vi "HFRR ADV v036 new software.vi"() -> ()   [LabVIEW 2025] (continued)
            n1884 = local write "Main Tab"(T2."Advance" ("Main Tab")) -> ()
            n1885 = local write "Main Dashboard Buttons"(T1."Advance" ("Main Dashboard Buttons")) -> ()
          }
        }
      }
    }
    n1886 = case shown="True" "Prog Uno" {
      frame False {
      }
      frame True {
        n1887 = stacked-sequence {
          frame #0 {
            n1888 = Delete(path (use dialog)=path "C:/LAB-IQ-NXT/UNOCOMPILE.bat" ("working directory")) -> ()  [unwired: 4 in, 3 out]
          }
          frame #1 {
            n1889 = local read "Com Port 1"() -> (w2647:refnum<visa-resource-name>)
            n1890 = Concatenate Strings("cmd.exe /c \"mode " ("command line"), w2647, ":1200,n,8,1\"\n" ("command line")) -> (w2652:string)
            n1891 = Concatenate Strings(w2652, "CD\\\nCD WinDucom\navrdude -C avrdude.conf -v -patmega328p -carduino -P" ("command line"), w2647, " -b115200 -D -Uflash:w:UNO_V20.hex:i\n" ("command line"), "\r") -> (w2654:string)
            "STR" <- w2654
            n1892 = call <vilib>:"Write Characters To File.vi"("append to file? (new file:F)"=FALSE, "character string"=w2654, "file path (dialog if empty)"=path "C:/LAB-IQ/UNOCOMPILE.bat" ("working directory")) -> ()  [unwired: 2 in, 1 out]
          }
          frame #2 {
            n1893 = disable-structure shown="Disabled" {
              frame Disabled {
                w2658 = "cmd.exe  /c \"C:\\LAB-IQ-NXT\\UNOCOMPILE.bat\"" ("string")
                n1894 = local write "Prog Uno"(FALSE ("run minimized? (F)")) -> ()
                n1895 = call <vilib>:"System Exec.vi"("expected output size  (4096)"=u32 65535, "run minimized? (F)"=FALSE, "wait until completion? (T)"=TRUE ("run minimized? (F)"), "working directory"=path "C:/LAB-IQ-NXT", "standard input"=w2658, "command line"=w2658) -> ("error out"=w2657:errorcluster, "standard output"=→"String 42":string)  [unwired: 2 in, 2 out]
                "error out 3" <- w2657
                n1896 = flat-sequence {
                  tunnel: w2657 -> [_]
                  frame #0 {
                  }
                }
              }
              frame Enabled {
              }
            }
          }
        }
      }
    }
    n1897 = case shown="\"ISO 12156\"" "TEST STANDARD" {
      frame "ASTM D6079", Default {
        w2627 = 50.0 ("Hz")
        w2628 = 53.0 ("Set Rh")
        w2630 = 1.0 ("Set Strk")
        w2629 = 60.0 ("Set Temp")
        # "astm hide"
        n1898 = local write "NORMAL LOAD"(200.0 ("NORMAL LOAD")) -> ()
        n1899 = local write "Set Strk"(w2630) -> ()
        n1900 = local write "Set Hz"(w2627) -> ()
        n1901 = local write "Set Temp"(w2629) -> ()
        n1902 = local write "Set Rh"(w2628) -> ()
        n1903 = local write "test time"(75.0 ("test time")) -> ()
        n1904 = local write "Set Stroke:"(w2630) -> ()
        n1905 = local write "Set Humidity:"(w2628) -> ()
        n1906 = local write "Set Frequency:"(w2627) -> ()
        n1907 = local write "Set Temperature:"(w2629) -> ()
        "Test Standard" <- "ASTM D6079" ("Test Standard 2")
      }
      frame "ISO 12156" {
        n1908 = local write "Set Strk"(1.0 ("Set Strk")) -> ()
        n1909 = local write "NORMAL LOAD"(200.0 ("NORMAL LOAD")) -> ()
        n1910 = local write "Set Temp"(60.0 ("Set Temp")) -> ()
        n1911 = local write "test time"(75.0 ("test time")) -> ()
        n1912 = local write "Set Hz"(50.0 ("Hz")) -> ()
        n1913 = local write "Set Rh"(53.0 ("Set Rh")) -> ()
      }
      frame "CEC F-096-A-06" {
        n1914 = local write "Set Strk"(1.0 ("Set Strk")) -> ()
        n1915 = local write "NORMAL LOAD"(200.0 ("NORMAL LOAD")) -> ()
        n1916 = local write "Set Temp"(60.0 ("Set Temp")) -> ()
        n1917 = local write "test time"(75.0 ("test time")) -> ()
        n1918 = local write "Set Hz"(50.0 ("Hz")) -> ()
        n1919 = local write "Set Rh"(53.0 ("Set Rh")) -> ()
      }
      frame "Custom" {
      }
    }
    n1920 = Or(x=w2180, y=w2178) -> (x .or. y?=w2179:bool)
    n1921 = case shown="\"About\"" w2177 {
      tunnel: [T28."Acquire" ("Main Tab") T28."Compare Files" ("Main Tab") T28."About" ("Main Tab")] -> w2188
      frame "Acquire", Default {
      }
      frame "Compare Files" {
      }
      frame "About" {
      }
    }
    n1922 = Or(x=w2183, y="OPEN") -> (x .or. y?=w2184:bool)
    n1923 = case shown="True" w2184 {
      tunnel: w2183 -> [_ w2216]
      frame False {
      }
      frame True {
        n1924 = stacked-sequence {
          tunnel: w2216 -> [_ w2283 _ _]
          frame #0 {
            w2232 = "  " ("String 6")
            n1925 = local write "OPEN"(FALSE ("open")) -> ()
            n1926 = local read "string1 2"() -> (w2220:string)
            n1927 = local read "string1 3"() -> (w2219:string)
            n1928 = local read "string1 4"() -> (w2218:string)
            n1929 = property on="OPEN" class="Bool (strict)"("Visible"=FALSE) -> ()  [unwired: 2 in, 2 out]
            n1930 = local write "String 6"(w2232) -> ()
            n1931 = local write "String 7"(w2232) -> ()
            n1932 = local write "String 8"(w2232) -> ()
            n1933 = local write "String 12"(w2232) -> ()
            n1934 = local read "OK Button 16"() -> (w2217:bool)
            n1935 = String To Path(string=w2220) -> (path=w2228:path)
            n1936 = String To Path(string=w2219) -> (path=w2227:path)
            n1937 = String To Path(string=w2218) -> (path=w2226:path)
            n1938 = case shown="True" w2217 {
              tunnel: [w2233 w2234] -> w2221
              frame False {
                n1939 = local read "string1"() -> (w2233:string)
              }
              frame True {
                n1940 = local read "String Indicator 4"() -> (w2234:string)
              }
            }
            n1941 = Open/Create/Replace File "Open File"(file path (use dialog)=w2228) -> (refnum out=w2224:refnum<file>)  [unwired: 5 in, 2 out]
            n1942 = Open/Create/Replace File "Open File"(file path (use dialog)=w2227) -> (refnum out=w2223:refnum<file>)  [unwired: 5 in, 2 out]
            n1943 = Open/Create/Replace File "Open File"(file path (use dialog)=w2226) -> (refnum out=w2222:refnum<file>)  [unwired: 5 in, 2 out]
            n1944 = while {
              tunnel: w2224 -> [w2246]
              i -> [w2242]
              stop <- w2241 continue-if-true
              (unwired) TRUE ("line mode (F)")
              n1945 = Read from Text File "Read File"(file (use dialog)=w2246) -> (text=w2243:string)  [unwired: 3 in, 3 out]
              n1946 = local write "Numeric 11"(w2242) -> ()
              n1947 = String Length(string=w2243) -> (length=w2245:i32)
              n1948 = Greater?(x=w2245, y=1) -> (0:w2241:bool)
            }
            n1949 = while {
              tunnel: w2223 -> [w2252]
              i -> [w2248]
              stop <- w2247 continue-if-true
              (unwired) TRUE ("line mode (F)")
              n1950 = Read from Text File "Read File"(file (use dialog)=w2252) -> (text=w2249:string)  [unwired: 3 in, 3 out]
              n1951 = local write "Numeric 12"(w2248) -> ()
              n1952 = String Length(string=w2249) -> (length=w2251:i32)
              n1953 = Greater?(x=w2251, y=1) -> (0:w2247:bool)
            }
            n1954 = while {
              tunnel: w2222 -> [w2258]
              i -> [w2254]
              stop <- w2253 continue-if-true
              (unwired) TRUE ("line mode (F)")
              n1955 = Read from Text File "Read File"(file (use dialog)=w2258) -> (text=w2255:string)  [unwired: 3 in, 3 out]
              n1956 = local write "Numeric 13"(w2254) -> ()
              n1957 = String Length(string=w2255) -> (length=w2257:i32)
              n1958 = Greater?(x=w2257, y=1) -> (0:w2253:bool)
            }
            n1959 = String To Path(string=w2221) -> (path=w2229:path)
            n1960 = Open/Create/Replace File "Open File"(file path (use dialog)=w2229) -> (refnum out=w2225:refnum<file>)  [unwired: 5 in, 2 out]
            n1961 = while {
              tunnel: w2225 -> [w2240]
              i -> [w2236]
              stop <- w2235 continue-if-true
              (unwired) TRUE ("line mode (F)")
              n1962 = Read from Text File "Read File"(file (use dialog)=w2240) -> (text=w2237:string)  [unwired: 3 in, 3 out]
              n1963 = local write "Numeric 8"(w2236) -> ()
              n1964 = String Length(string=w2237) -> (length=w2239:i32)
              n1965 = Greater?(x=w2239, y=1) -> (0:w2235:bool)
            }
          }
          frame #1 {
            w2410 = FALSE ("ACTUAL   MERGE")
            # "Sample Temp"
            # "ECR"
            # "COF"
            # "Time\nCOF\nFF\nTemp"
            n1966 = case shown="True" w2283 {
              tunnel: [w2430 w2431] -> w2284
              frame False {
                n1967 = local read "string1"() -> (w2430:string)
              }
              frame True {
                n1968 = local read "String Indicator 4"() -> (w2431:string)
              }
            }
            n1969 = local read "string1 3"() -> (w2328:string)
            n1970 = String To Path(string=w2284) -> (path=w2415:path)
            n1971 = String To Path(string=w2328) -> (path=w2426:path)
            n1972 = local read "Numeric 12"() -> (w2412:i32)
            n1973 = local read "Numeric 8"() -> (w2414:i32)
            n1974 = local read "string1 2"() -> (w2329:string)
            n1975 = local read "string1 4"() -> (w2327:string)
            n1976 = Open/Create/Replace File "Open File"(file path (use dialog)=w2415) -> (refnum out=w2429:refnum<file>, error out=w2428:errorcluster)  [unwired: 5 in, 1 out]
            n1977 = Open/Create/Replace File "Open File"(file path (use dialog)=w2426) -> (refnum out=w2422:refnum<file>, error out=w2423:errorcluster)  [unwired: 5 in, 1 out]
            n1978 = for {
              N: w2414 -> [_]
              tunnel: w2429 -> [w2577]
              tunnel: w2428 -> [w2576]
              tunnel: [w2566] -> w2341 mode=indexing
              tunnel: [w2564] -> w2398 mode=indexing
              tunnel: [w2565] -> w2393 mode=indexing
              tunnel: w2410 -> [_]
              tunnel: [w2558] -> w2395 mode=indexing
              tunnel: [w2554] -> w2364 mode=indexing
              tunnel: [w2550] -> w2339 mode=indexing
              tunnel: [w2546] -> w2320 mode=indexing
              tunnel: [w2541] -> w2280 mode=indexing
              (unwired) TRUE ("line mode (F)")
              # "freq"
              # "Stroke"
              # "Time"
              # "CoF"
              # "Humidity"
              # "Temp"
              # "Air Temp"
              # "ECR"
              n1979 = Read from Text File "Read File"(file (use dialog)=w2577, error in=w2576) -> (text=w2542:string)  [unwired: 2 in, 3 out]
              n1980 = local write "String 6"(w2542) -> ()
              n1981 = String Subset(string=w2542, offset (0)=0, length (rest)=14 ("length (rest)")) -> (substring=w2570:string)
              n1982 = String Subset(string=w2542, offset (0)=35, length (rest)=9 ("length (rest)")) -> (substring=w2567:string)
              n1983 = String Subset(string=w2542, offset (0)=15, length (rest)=9 ("length (rest)")) -> (substring=w2573:string)
              n1984 = Fract/Exp String To Number(string=w2570) -> (number=w2566:dbl)  [unwired: 3 in, 1 out]
              n1985 = Fract/Exp String To Number(string=w2567) -> (number=w2565:dbl)  [unwired: 3 in, 1 out]
              n1986 = Fract/Exp String To Number(string=w2573) -> (number=w2564:dbl)  [unwired: 3 in, 1 out]
              n1987 = String Subset(string=w2542, offset (0)=85, length (rest)=9 ("length (rest)")) -> (substring=w2543:string)
              n1988 = String Subset(string=w2542, offset (0)=25, length (rest)=9 ("length (rest)")) -> (substring=w2549:string)
              n1989 = String Subset(string=w2542, offset (0)=55, length (rest)=9 ("length (rest)")) -> (substring=w2551:string)
              n1990 = String Subset(string=w2542, offset (0)=45, length (rest)=9 ("length (rest)")) -> (substring=w2557:string)
              n1991 = String Subset(string=w2542, offset (0)=65, length (rest)=9 ("length (rest)")) -> (substring=w2563:string)
              n1992 = Fract/Exp String To Number(string=w2549) -> (number=w2546:dbl)  [unwired: 3 in, 1 out]
              n1993 = Fract/Exp String To Number(string=w2543) -> (number=w2541:dbl)  [unwired: 3 in, 1 out]
              n1994 = Fract/Exp String To Number(string=w2551) -> (number=w2550:dbl)  [unwired: 3 in, 1 out]
              n1995 = Fract/Exp String To Number(string=w2557) -> (number=w2554:dbl)  [unwired: 3 in, 1 out]
              n1996 = Fract/Exp String To Number(string=w2563) -> (number=w2560:dbl)  [unwired: 3 in, 1 out]
              n1997 = Add(x=w2560, y=0.0) -> (x+y=w2558:dbl)
            }
            n1998 = for {
              N: w2412 -> [_]
              tunnel: w2423 -> [w2503]
              tunnel: w2422 -> [w2502]
              tunnel: [w2492] -> w2381 mode=indexing
              tunnel: [w2490] -> w2379 mode=indexing
              tunnel: [w2491] -> w2375 mode=indexing
              tunnel: w2410 -> [_]
              tunnel: [w2484] -> w2377 mode=indexing
              tunnel: [w2480] -> w2359 mode=indexing
              tunnel: [w2476] -> w2335 mode=indexing
              tunnel: [w2473] -> w2316 mode=indexing
              tunnel: [w2469] -> w2275 mode=indexing
              (unwired) 9 ("length (rest)")
              (unwired) 9 ("length (rest)")
              (unwired) TRUE ("line mode (F)")
              n1999 = Read from Text File "Read File"(file (use dialog)=w2502, error in=w2503) -> (text=w2470:string)  [unwired: 2 in, 3 out]
              n2000 = local write "String 8"(w2470) -> ()
              n2001 = String Subset(string=w2470, offset (0)=85) -> (substring=w2472:string)  [unwired: 1 in]
              n2002 = String Subset(string=w2470, offset (0)=35, length (rest)=9 ("length (rest)")) -> (substring=w2493:string)
              n2003 = String Subset(string=w2470, offset (0)=55, length (rest)=9 ("length (rest)")) -> (substring=w2478:string)
              n2004 = String Subset(string=w2470, offset (0)=25) -> (substring=w2474:string)  [unwired: 1 in]
              n2005 = String Subset(string=w2470, offset (0)=15, length (rest)=9 ("length (rest)")) -> (substring=w2499:string)
              n2006 = String Subset(string=w2470, offset (0)=0, length (rest)=14 ("length (rest)")) -> (substring=w2496:string)
              n2007 = String Subset(string=w2470, offset (0)=45, length (rest)=9 ("length (rest)")) -> (substring=w2483:string)
              n2008 = String Subset(string=w2470, offset (0)=65, length (rest)=9 ("length (rest)")) -> (substring=w2489:string)
              n2009 = Fract/Exp String To Number(string=w2472) -> (number=w2469:dbl)  [unwired: 3 in, 1 out]
              n2010 = Fract/Exp String To Number(string=w2493) -> (number=w2491:dbl)  [unwired: 3 in, 1 out]
              n2011 = Fract/Exp String To Number(string=w2478) -> (number=w2476:dbl)  [unwired: 3 in, 1 out]
              n2012 = Fract/Exp String To Number(string=w2474) -> (number=w2473:dbl)  [unwired: 3 in, 1 out]
              n2013 = Fract/Exp String To Number(string=w2499) -> (number=w2490:dbl)  [unwired: 3 in, 1 out]
              n2014 = Fract/Exp String To Number(string=w2496) -> (number=w2492:dbl)  [unwired: 3 in, 1 out]
              n2015 = Fract/Exp String To Number(string=w2483) -> (number=w2480:dbl)  [unwired: 3 in, 1 out]
              n2016 = Fract/Exp String To Number(string=w2489) -> (number=w2486:dbl)  [unwired: 3 in, 1 out]
              n2017 = Add(x=w2486, y=0.0) -> (x+y=w2484:dbl)
            }
            n2018 = String To Path(string=w2329) -> (path=w2427:path)
            n2019 = String To Path(string=w2327) -> (path=w2421:path)
            n2020 = local read "Numeric 11"() -> (w2411:i32)
            n2021 = local read "Numeric 13"() -> (w2413:i32)
            n2022 = Open/Create/Replace File "Open File"(file path (use dialog)=w2427) -> (refnum out=w2425:refnum<file>, error out=w2424:errorcluster)  [unwired: 5 in, 1 out]
            n2023 = Open/Create/Replace File "Open File"(file path (use dialog)=w2421) -> (refnum out=w2420:refnum<file>, error out=w2419:errorcluster)  [unwired: 5 in, 1 out]
            n2024 = for {
              N: w2411 -> [_]
              tunnel: w2425 -> [w2540]
              tunnel: w2424 -> [w2539]
              tunnel: [w2529] -> w2391 mode=indexing
              tunnel: [w2527] -> w2389 mode=indexing
              tunnel: [w2528] -> w2384 mode=indexing
              tunnel: w2410 -> [_]
              tunnel: [w2521] -> w2386 mode=indexing
              tunnel: [w2517] -> w2362 mode=indexing
              tunnel: [w2513] -> w2337 mode=indexing
              tunnel: [w2509] -> w2318 mode=indexing
              tunnel: [w2504] -> w2276 mode=indexing
              (unwired) TRUE ("line mode (F)")
              n2025 = Read from Text File "Read File"(file (use dialog)=w2540, error in=w2539) -> (text=w2505:string)  [unwired: 2 in, 3 out]
              n2026 = local write "String 7"(w2505) -> ()
              n2027 = String Subset(string=w2505, offset (0)=85, length (rest)=9 ("length (rest)")) -> (substring=w2508:string)
              n2028 = String Subset(string=w2505, offset (0)=35, length (rest)=9 ("length (rest)")) -> (substring=w2530:string)
              n2029 = String Subset(string=w2505, offset (0)=55, length (rest)=9 ("length (rest)")) -> (substring=w2516:string)
              n2030 = String Subset(string=w2505, offset (0)=25, length (rest)=9 ("length (rest)")) -> (substring=w2510:string)
              n2031 = String Subset(string=w2505, offset (0)=45, length (rest)=9 ("length (rest)")) -> (substring=w2518:string)
              n2032 = String Subset(string=w2505, offset (0)=0, length (rest)=14 ("length (rest)")) -> (substring=w2533:string)
              n2033 = String Subset(string=w2505, offset (0)=15, length (rest)=9 ("length (rest)")) -> (substring=w2536:string)
              n2034 = String Subset(string=w2505, offset (0)=65, length (rest)=9 ("length (rest)")) -> (substring=w2522:string)
              n2035 = Fract/Exp String To Number(string=w2508) -> (number=w2504:dbl)  [unwired: 3 in, 1 out]
              n2036 = Fract/Exp String To Number(string=w2530) -> (number=w2528:dbl)  [unwired: 3 in, 1 out]
              n2037 = Fract/Exp String To Number(string=w2516) -> (number=w2513:dbl)  [unwired: 3 in, 1 out]
              n2038 = Fract/Exp String To Number(string=w2510) -> (number=w2509:dbl)  [unwired: 3 in, 1 out]
              n2039 = Fract/Exp String To Number(string=w2518) -> (number=w2517:dbl)  [unwired: 3 in, 1 out]
              n2040 = Fract/Exp String To Number(string=w2533) -> (number=w2529:dbl)  [unwired: 3 in, 1 out]
              n2041 = Fract/Exp String To Number(string=w2536) -> (number=w2527:dbl)  [unwired: 3 in, 1 out]
              n2042 = Fract/Exp String To Number(string=w2522) -> (number=w2525:dbl)  [unwired: 3 in, 1 out]
              n2043 = Add(x=w2525, y=0.0) -> (x+y=w2521:dbl)
            }
            n2044 = for {
              N: w2413 -> [_]
              tunnel: w2420 -> [w2468]
              tunnel: w2419 -> [w2467]
              tunnel: [w2457] -> w2373 mode=indexing
              tunnel: [w2456] -> w2366 mode=indexing
              tunnel: w2410 -> [_]
              tunnel: [w2445] -> w2371 mode=indexing
              tunnel: [w2450] -> w2368 mode=indexing
              tunnel: [w2446] -> w2358 mode=indexing
              tunnel: [w2441] -> w2333 mode=indexing
              tunnel: [w2437] -> w2314 mode=indexing
              tunnel: [w2432] -> w2274 mode=indexing
              (unwired) 1.0 ("x")
              (unwired) TRUE ("line mode (F)")
              n2045 = Read from Text File "Read File"(file (use dialog)=w2468, error in=w2467) -> (text=w2433:string)  [unwired: 2 in, 3 out]
              n2046 = local write "String 12"(w2433) -> ()
              n2047 = String Subset(string=w2433, offset (0)=85, length (rest)=9 ("length (rest)")) -> (substring=w2435:string)
              n2048 = String Subset(string=w2433, offset (0)=35, length (rest)=9 ("length (rest)")) -> (substring=w2458:string)
              n2049 = String Subset(string=w2433, offset (0)=55, length (rest)=9 ("length (rest)")) -> (substring=w2443:string)
              n2050 = String Subset(string=w2433, offset (0)=25, length (rest)=9 ("length (rest)")) -> (substring=w2439:string)
              n2051 = String Subset(string=w2433, offset (0)=45, length (rest)=9 ("length (rest)")) -> (substring=w2448:string)
              n2052 = String Subset(string=w2433, offset (0)=15, length (rest)=9 ("length (rest)")) -> (substring=w2464:string)
              n2053 = String Subset(string=w2433, offset (0)=0, length (rest)=14 ("length (rest)")) -> (substring=w2461:string)
              n2054 = String Subset(string=w2433, offset (0)=65, length (rest)=9 ("length (rest)")) -> (substring=w2451:string)
              n2055 = Fract/Exp String To Number(string=w2435) -> (number=w2432:dbl)  [unwired: 3 in, 1 out]
              n2056 = Fract/Exp String To Number(string=w2458) -> (number=w2456:dbl)  [unwired: 3 in, 1 out]
              n2057 = Fract/Exp String To Number(string=w2443) -> (number=w2441:dbl)  [unwired: 3 in, 1 out]
              n2058 = Fract/Exp String To Number(string=w2439) -> (number=w2437:dbl)  [unwired: 3 in, 1 out]
              n2059 = Fract/Exp String To Number(string=w2448) -> (number=w2446:dbl)  [unwired: 3 in, 1 out]
              n2060 = Fract/Exp String To Number(string=w2464) -> (number=w2445:dbl)  [unwired: 3 in, 1 out]
              n2061 = Fract/Exp String To Number(string=w2461) -> (number=w2457:dbl)  [unwired: 3 in, 1 out]
              n2062 = Fract/Exp String To Number(string=w2451) -> (number=w2454:dbl)  [unwired: 3 in, 1 out]
              n2063 = Add(x=w2454, y=0.0) -> (x+y=w2450:dbl)
            }
            n2064 = Delete From Array(array=w2316, index=0) -> (array with subset deleted=w2289:dbl[])  [unwired: 1 in, 1 out]
            n2065 = Delete From Array(array=w2379, index=0) -> (array with subset deleted=w2352:dbl[])  [unwired: 1 in, 1 out]
            n2066 = Delete From Array(array=w2359, index=0) -> (array with subset deleted=w2347:dbl[])  [unwired: 1 in, 1 out]
            n2067 = Delete From Array(array=w2377, index=0) -> (array with subset deleted=w2378:dbl[])  [unwired: 1 in, 1 out]
            n2068 = call-poly <vilib>:"Mean.vi"("X"=w2289) -> ("mean"=→"КОФ2 4":dbl)  [unwired: 1 out]
            n2069 = call-poly <vilib>:"Mean.vi"("X"=w2352) -> ("mean"=→"КОФ3":dbl)  [unwired: 1 out]
            n2070 = call-poly <vilib>:"Mean.vi"("X"=w2347) -> ("mean"=→"CP3":dbl)  [unwired: 1 out]
            n2071 = Delete From Array(array=w2341, index=0) -> (array with subset deleted=w2268:dbl[])  [unwired: 1 in, 1 out]
            n2072 = Delete From Array(array=w2280, index=0) -> (array with subset deleted=w2267:dbl[])  [unwired: 1 in, 1 out]
            n2073 = Delete From Array(array=w2320, index=0) -> (array with subset deleted=w2291:dbl[])  [unwired: 1 in, 1 out]
            n2074 = Delete From Array(array=w2398, index=0) -> (array with subset deleted=w2353:dbl[])  [unwired: 1 in, 1 out]
            n2075 = Delete From Array(array=w2364, index=0) -> (array with subset deleted=w2349:dbl[])  [unwired: 1 in, 1 out]
            "array w/ subset deleted" <- w2349
            n2076 = Delete From Array(array=w2395, index=0) -> (array with subset deleted=w2396:dbl[])  [unwired: 1 in, 1 out]
            n2077 = call-poly <vilib>:"Mean.vi"("X"=w2291) -> ("mean"=→"КОФ2 2":dbl)  [unwired: 1 out]
            n2078 = call-poly <vilib>:"Mean.vi"("X"=w2353) -> ("mean"=→"КОФ1":dbl)  [unwired: 1 out]
            n2079 = Bundle "Bundle"(w2268, w2267) -> (w2273:cluster{dbl[], dbl[]})  [unwired: 1 in]
            n2080 = Bundle "Bundle"(w2268, w2396) -> (w2260:cluster{dbl[], dbl[]})  [unwired: 1 in]
            n2081 = Delete From Array(array=w2275, index=0) -> (array with subset deleted=w2263:dbl[])  [unwired: 1 in, 1 out]
            n2082 = Delete From Array(array=w2276, index=0) -> (array with subset deleted=w2265:dbl[])  [unwired: 1 in, 1 out]
            n2083 = Delete From Array(array=w2386, index=0) -> (array with subset deleted=w2387:dbl[])  [unwired: 1 in, 1 out]
            n2084 = Delete From Array(array=w2274, index=0) -> (array with subset deleted=w2261:dbl[])  [unwired: 1 in, 1 out]
            n2085 = Delete From Array(array=w2368, index=0) -> (array with subset deleted=w2369:dbl[])  [unwired: 1 in, 1 out]
            n2086 = Delete From Array(array=w2393, index=0) -> (array with subset deleted=w2299:dbl[])  [unwired: 1 in, 1 out]
            n2087 = Delete From Array(array=w2339, index=0) -> (array with subset deleted=w2295:dbl[])  [unwired: 1 in, 1 out]
            n2088 = Delete From Array(array=w2375, index=0) -> (array with subset deleted=w2297:dbl[])  [unwired: 1 in, 1 out]
            n2089 = Delete From Array(array=w2335, index=0) -> (array with subset deleted=w2293:dbl[])  [unwired: 1 in, 1 out]
            n2090 = Delete From Array(array=w2384, index=0) -> (array with subset deleted=w2298:dbl[])  [unwired: 1 in, 1 out]
            n2091 = Delete From Array(array=w2337, index=0) -> (array with subset deleted=w2294:dbl[])  [unwired: 1 in, 1 out]
            n2092 = Delete From Array(array=w2318, index=0) -> (array with subset deleted=w2290:dbl[])  [unwired: 1 in, 1 out]
            n2093 = Delete From Array(array=w2362, index=0) -> (array with subset deleted=w2348:dbl[])  [unwired: 1 in, 1 out]
            n2094 = Delete From Array(array=w2389, index=0) -> (array with subset deleted=w2350:dbl[])  [unwired: 1 in, 1 out]
            n2095 = Delete From Array(array=w2366, index=0) -> (array with subset deleted=w2296:dbl[])  [unwired: 1 in, 1 out]
            n2096 = Delete From Array(array=w2333, index=0) -> (array with subset deleted=w2292:dbl[])  [unwired: 1 in, 1 out]
            n2097 = Delete From Array(array=w2314, index=0) -> (array with subset deleted=w2288:dbl[])  [unwired: 1 in, 1 out]
            n2098 = Delete From Array(array=w2358, index=0) -> (array with subset deleted=w2346:dbl[])  [unwired: 1 in, 1 out]
            n2099 = Delete From Array(array=w2371, index=0) -> (array with subset deleted=w2351:dbl[])  [unwired: 1 in, 1 out]
            n2100 = Delete From Array(array=w2381, index=0) -> (array with subset deleted=w2264:dbl[])  [unwired: 1 in, 1 out]
            n2101 = Delete From Array(array=w2391, index=0) -> (array with subset deleted=w2266:dbl[])  [unwired: 1 in, 1 out]
            n2102 = Delete From Array(array=w2373, index=0) -> (array with subset deleted=w2262:dbl[])  [unwired: 1 in, 1 out]
            n2103 = Bundle "Bundle"(w2268, w2299) -> (w2286:cluster{dbl[], dbl[]})  [unwired: 1 in]
            n2104 = Bundle "Bundle"(w2268, w2353) -> (w2287:cluster{dbl[], dbl[]})  [unwired: 1 in]
            n2105 = Bundle "Bundle"(w2299, w2295) -> (w2301:cluster{dbl[], dbl[]})  [unwired: 1 in]
            n2106 = Bundle "Bundle"(w2264, w2263) -> (w2271:cluster{dbl[], dbl[]})  [unwired: 1 in]
            n2107 = Bundle "Bundle"(w2297, w2293) -> (w2303:cluster{dbl[], dbl[]})  [unwired: 1 in]
            n2108 = Bundle "Bundle"(w2264, w2297) -> (w2407:cluster{dbl[], dbl[]})  [unwired: 1 in]
            n2109 = Bundle "Bundle"(w2264, w2293) -> (w2331:cluster{dbl[], dbl[]})  [unwired: 1 in]
            n2110 = Bundle "Bundle"(w2264, w2352) -> (w2417:cluster{dbl[], dbl[]})  [unwired: 1 in]
            n2111 = Bundle "Bundle"(w2264, w2347) -> (w2355:cluster{dbl[], dbl[]})  [unwired: 1 in]
            n2112 = Bundle "Bundle"(w2264, w2378) -> (w2402:cluster{dbl[], dbl[]})  [unwired: 1 in]
            n2113 = Bundle "Bundle"(w2298, w2294) -> (w2302:cluster{dbl[], dbl[]})  [unwired: 1 in]
            n2114 = Bundle "Bundle"(w2266, w2265) -> (w2272:cluster{dbl[], dbl[]})  [unwired: 1 in]
            n2115 = Bundle "Bundle"(w2266, w2298) -> (w2409:cluster{dbl[], dbl[]})  [unwired: 1 in]
            n2116 = Bundle "Bundle"(w2266, w2294) -> (w2332:cluster{dbl[], dbl[]})  [unwired: 1 in]
            n2117 = Bundle "Bundle"(w2266, w2348) -> (w2356:cluster{dbl[], dbl[]})  [unwired: 1 in]
            n2118 = Bundle "Bundle"(w2266, w2350) -> (w2418:cluster{dbl[], dbl[]})  [unwired: 1 in]
            n2119 = Bundle "Bundle"(w2266, w2387) -> (w2400:cluster{dbl[], dbl[]})  [unwired: 1 in]
            n2120 = Bundle "Bundle"(w2296, w2292) -> (w2304:cluster{dbl[], dbl[]})  [unwired: 1 in]
            n2121 = Bundle "Bundle"(w2262, w2261) -> (w2270:cluster{dbl[], dbl[]})  [unwired: 1 in]
            n2122 = Bundle "Bundle"(w2262, w2296) -> (w2408:cluster{dbl[], dbl[]})  [unwired: 1 in]
            n2123 = Bundle "Bundle"(w2262, w2292) -> (w2330:cluster{dbl[], dbl[]})  [unwired: 1 in]
            n2124 = Bundle "Bundle"(w2262, w2346) -> (w2354:cluster{dbl[], dbl[]})  [unwired: 1 in]
            n2125 = Bundle "Bundle"(w2262, w2351) -> (w2416:cluster{dbl[], dbl[]})  [unwired: 1 in]
            n2126 = Bundle "Bundle"(w2262, w2369) -> (w2401:cluster{dbl[], dbl[]})  [unwired: 1 in]
            n2127 = call-poly <vilib>:"Mean.vi"("X"=w2349) -> ("mean"=→"CP1":dbl)  [unwired: 1 out]
            n2128 = call-poly <vilib>:"Mean.vi"("X"=w2290) -> ("mean"=→"КОФ2 3":dbl)  [unwired: 1 out]
            n2129 = call-poly <vilib>:"Mean.vi"("X"=w2348) -> ("mean"=→"CP2":dbl)  [unwired: 1 out]
            n2130 = call-poly <vilib>:"Mean.vi"("X"=w2350) -> ("mean"=→"КОФ2":dbl)  [unwired: 1 out]
            n2131 = call-poly <vilib>:"Mean.vi"("X"=w2288) -> ("mean"=→"КОФ2 5":dbl)  [unwired: 1 out]
            n2132 = call-poly <vilib>:"Mean.vi"("X"=w2346) -> ("mean"=→"CP4":dbl)  [unwired: 1 out]
            n2133 = call-poly <vilib>:"Mean.vi"("X"=w2351) -> ("mean"=→"КОФ4":dbl)  [unwired: 1 out]
            n2134 = Bundle "Bundle"(w2268, w2295) -> (w2259:cluster{dbl[], dbl[]})  [unwired: 1 in]
            n2135 = Bundle "Bundle"(w2268, w2349) -> (w2282:cluster{dbl[], dbl[]})  [unwired: 1 in]
            n2136 = Build Array "Build Array"(w2259, w2282) -> (w2285:cluster{dbl[], dbl[]}[])
            "XY Graph 17" <- w2285
            n2137 = Build Array "Build Array"(w2273, w2272, w2271, w2270) -> (→"Frequency ( Hz )":cluster{dbl[], dbl[]}[])
            n2138 = Build Array "Build Array"(w2301, w2302, w2303, w2304) -> (→"Air Temp ( °C ) vs Humidity ( % RH )":cluster{dbl[], dbl[]}[])
            n2139 = Build Array "Build Array"(w2286, w2409, w2407, w2408) -> (→"Air Temperature  ( °C )":cluster{dbl[], dbl[]}[])
            n2140 = Build Array "Build Array"(w2259, w2332, w2331, w2330) -> (→"Humidity ( %RH )":cluster{dbl[], dbl[]}[])
            n2141 = Build Array "Build Array"(w2287, w2418, w2417, w2416) -> (→"Coefficient Of Friction":cluster{dbl[], dbl[]}[])
            n2142 = Build Array "Build Array"(w2282, w2356, w2355, w2354) -> (→"Sample Temperature ( °C )":cluster{dbl[], dbl[]}[])
            n2143 = Build Array "Build Array"(w2260, w2400, w2402, w2401) -> (→"XY Graph 13":cluster{dbl[], dbl[]}[])
            n2144 = Bundle "Bundle"(w2268, w2291) -> (w2313:cluster{dbl[], dbl[]})  [unwired: 1 in]
            n2145 = Bundle "Bundle"(w2264, w2289) -> (w2311:cluster{dbl[], dbl[]})  [unwired: 1 in]
            n2146 = Bundle "Bundle"(w2266, w2290) -> (w2312:cluster{dbl[], dbl[]})  [unwired: 1 in]
            n2147 = Bundle "Bundle"(w2262, w2288) -> (w2310:cluster{dbl[], dbl[]})  [unwired: 1 in]
            n2148 = Build Array "Build Array"(w2313, w2312, w2311, w2310) -> (→"Stroke ( mm )":cluster{dbl[], dbl[]}[])
            n2149 = local write "XY Graph 16"(w2285) -> ()
          }
          frame #2 {
          }
          frame #3 {
            n2150 = local write "Numeric 8"(0 ("Numeric 8")) -> ()
            n2151 = local write "Numeric 11"(0 ("Numeric 11")) -> ()
            n2152 = local write "Numeric 12"(0 ("Numeric 12")) -> ()
            n2153 = local write "Numeric 13"(0 ("Numeric 13")) -> ()
            n2154 = property on="OPEN" class="Bool (strict)"("Visible"=TRUE) -> ()  [unwired: 2 in, 2 out]
            n2155 = local read "String Control 2"() -> (w2585:string)
            n2156 = local read "String Control 4"() -> (w2584:string)
            n2157 = local read "String Control 6"() -> (w2583:string)
            n2158 = local read "String Control 8"() -> (w2582:string)
            n2159 = Match Pattern(string=w2585, regular expression="Samples / cycle :- ") -> (after substring=w2599:string)  [unwired: 1 in, 3 out]
            n2160 = Match Pattern(string=w2585, regular expression="Frequency :- ") -> (after substring=w2618:string)  [unwired: 1 in, 3 out]
            n2161 = Match Pattern(string=w2584, regular expression="Samples / cycle :- ") -> (after substring=w2595:string)  [unwired: 1 in, 3 out]
            n2162 = Match Pattern(string=w2584, regular expression="Frequency :- ") -> (after substring=w2613:string)  [unwired: 1 in, 3 out]
            n2163 = Match Pattern(string=w2583, regular expression="Samples / cycle :- ") -> (after substring=w2591:string)  [unwired: 1 in, 3 out]
            n2164 = Match Pattern(string=w2583, regular expression="Frequency :- ") -> (after substring=w2608:string)  [unwired: 1 in, 3 out]
            n2165 = Match Pattern(string=w2582, regular expression="Samples / cycle :- ") -> (after substring=w2587:string)  [unwired: 1 in, 3 out]
            n2166 = Match Pattern(string=w2582, regular expression="Frequency :- ") -> (after substring=w2603:string)  [unwired: 1 in, 3 out]
            n2167 = String Subset(string=w2599, length (rest)=6 ("length (rest)")) -> (substring=w2601:string)  [unwired: 1 in]
            n2168 = String Subset(string=w2618, length (rest)=9 ("length (rest)")) -> (substring=w2620:string)  [unwired: 1 in]
            n2169 = String Subset(string=w2595, length (rest)=6 ("length (rest)")) -> (substring=w2597:string)  [unwired: 1 in]
            n2170 = String Subset(string=w2613, length (rest)=9 ("length (rest)")) -> (substring=w2615:string)  [unwired: 1 in]
            n2171 = String Subset(string=w2591, length (rest)=6 ("length (rest)")) -> (substring=w2593:string)  [unwired: 1 in]
            n2172 = String Subset(string=w2608, length (rest)=9 ("length (rest)")) -> (substring=w2610:string)  [unwired: 1 in]
            n2173 = String Subset(string=w2587, length (rest)=6 ("length (rest)")) -> (substring=w2589:string)  [unwired: 1 in]
            n2174 = String Subset(string=w2603, length (rest)=9 ("length (rest)")) -> (substring=w2605:string)  [unwired: 1 in]
            n2175 = Fract/Exp String To Number(string=w2601) -> (number=w2581:dbl)  [unwired: 3 in, 1 out]
            n2176 = Fract/Exp String To Number(string=w2620) -> (number=w2621:dbl)  [unwired: 3 in, 1 out]
            n2177 = Fract/Exp String To Number(string=w2597) -> (number=w2580:dbl)  [unwired: 3 in, 1 out]
            n2178 = Fract/Exp String To Number(string=w2615) -> (number=w2616:dbl)  [unwired: 3 in, 1 out]
            n2179 = Fract/Exp String To Number(string=w2593) -> (number=w2579:dbl)  [unwired: 3 in, 1 out]
            n2180 = Fract/Exp String To Number(string=w2610) -> (number=w2611:dbl)  [unwired: 3 in, 1 out]
            n2181 = Fract/Exp String To Number(string=w2589) -> (number=w2578:dbl)  [unwired: 3 in, 1 out]
            n2182 = Fract/Exp String To Number(string=w2605) -> (number=w2606:dbl)  [unwired: 3 in, 1 out]
            n2183 = local write "sample1"(w2581) -> ()
            n2184 = local write "freq1"(w2621) -> ()
            n2185 = local write "sample2"(w2580) -> ()
            n2186 = local write "freq2"(w2616) -> ()
            n2187 = local write "sample3"(w2579) -> ()
            n2188 = local write "freq3"(w2611) -> ()
            n2189 = local write "sample4"(w2578) -> ()
            n2190 = local write "freq 4"(w2606) -> ()
          }
        }
      }
    }
    n2191 = case shown="True" w2179 {
      selector: w2179 -> [_ w2198]
      frame False {
      }
      frame True {
        n2192 = Not(x=w2198) -> (.not. x?=w2194:bool)
        n2193 = local write "service 3"(w2194) -> ()
        n2194 = local write "OPEN 6"(w2194) -> ()
        n2195 = call <vilib>:"System Exec.vi"("wait until completion? (T)"=TRUE, "command line"="C:\\LAB-IQ\\Scar View.exe") -> ("error out"=→"error out 5":errorcluster)  [unwired: 6 in, 3 out]
      }
    }
    n2196 = case shown="\"Acquire\", Default" w2188 {
      frame "Acquire", Default {
        # "Elapsed time\ncof\nstroke\nAir temp\nTemp\nHumidity"
        n2197 = disable-structure shown="Disabled" {
          frame Disabled {
            n2198 = local read "Flag"() -> (w2897:dbl)
            n2199 = local read "RUN"() -> (w2894:bool)
            n2200 = Not(x=w2894) -> (.not. x?=w2893:bool)
            n2201 = Equal?(x=w2897, y=10.0) -> (x = y?=w2895:bool)
            n2202 = And(x=w2895, y=w2893) -> (x .and. y?=w2892:bool)
            n2203 = case shown="True" w2892 {
              frame False {
              }
              frame True {
                w2898 = FALSE ("Heater Button")
                n2204 = local write "Humidity"(w2898) -> ()
                n2205 = local write "Heater Button"(w2898) -> ()
              }
            }
          }
          frame Enabled {
          }
        }
        n2206 = disable-structure shown="Disabled" {
          frame Disabled {
            n2207 = case shown="True" {
              selector: _ -> [_ _]
              frame False {
              }
              frame True {
                w2947 = TRUE ("Heater")
                n2208 = local write "Humidity"(w2947) -> ()
                n2209 = local write "Heater Button"(w2947) -> ()
                n2210 = local read "TEST STANDARD"() -> (w2950:T3)
                n2211 = local read "TEST STANDARD"() -> (w2945:T3)
                n2212 = Equal?(x=w2950, y=enum16{"ASTM D6079", "ISO 12156", "Custom"}."ISO 12156" ("Test Standard")) -> (x = y?=w2948:bool)
                n2213 = Equal?(x=w2945, y=enum16{"ASTM D6079", "ISO 12156", "Custom"}."ASTM D6079" ("Test Standard")) -> (x = y?=w2944:bool)
                n2214 = case shown="True" w2948 {
                  frame False {
                  }
                  frame True {
                    n2215 = local write "airtempflg"(FALSE ("airtempflg")) -> ()
                    n2216 = local write item#-1(TRUE ("Heater")) -> ()
                  }
                }
                n2217 = case shown="True" w2944 {
                  frame False {
                  }
                  frame True {
                    n2218 = local write "airtempflg"(TRUE ("airtempflg")) -> ()
                    n2219 = local write item#-1(FALSE ("Heater")) -> ()
                  }
                }
              }
            }
          }
          frame Enabled {
          }
        }
        n2220 = stacked-sequence {
          frame #0 {
            n2221 = case shown="True" "RST FF" {
              frame False {
              }
              frame True {
                w2964 = 0.0 ("X Scale.Range:Maximum")
                n2222 = property on="Frictional Force ( N )" class="WFChart (strict)"("XScale.Maximum"=600.0 ("X Scale.Range:Maximum"), "XScale.Minimum"=w2964, "YScale.Maximum"=10.0 ("Y Scale.Range:Maximum"), "YScale.Minimum"=w2964) -> ()  [unwired: 2 in, 2 out]
              }
            }
          }
          frame #1 {
            n2223 = case shown="True" "RST TEMP" {
              frame False {
              }
              frame True {
                n2224 = property on="Temperature ( Deg C )" class="WFChart (strict)"("XScale.Minimum"=0.0 ("X Scale.Range:Minimum"), "XScale.Maximum"=600.0 ("X Scale.Range:Maximum"), "YScale.Minimum"=0.0 ("Y Scale.Range:Minimum"), "YScale.Maximum"=100.0 ("Y Scale.Range:Maximum")) -> ()  [unwired: 2 in, 2 out]
              }
            }
          }
          frame #2 {
            n2225 = case shown="True" "RSTCOF" {
              frame False {
              }
              frame True {
                n2226 = property on="Coefficient of Friction" class="WFChart (strict)"("XScale.Minimum"=0.0 ("X Scale.Range:Minimum"), "XScale.Maximum"=600.0 ("X Scale.Range:Maximum"), "YScale.Maximum"=1.0 ("X Scale.Range:Minimum"), "YScale.Minimum"=0.0 ("X Scale.Range:Minimum")) -> ()  [unwired: 2 in, 2 out]
              }
            }
          }
          frame #3 {
            n2227 = case shown="True" "RSTCOF 2" {
              frame False {
              }
              frame True {
                (unwired) 100.0 ("Y Scale.Range:Maximum")
                (unwired) 0.0 ("Y Scale.Range:Minimum")
                (unwired) 600.0 ("X Scale.Range:Maximum")
                (unwired) 0.0 ("X Scale.Range:Minimum")
              }
            }
          }
          frame #4 {
            n2228 = case shown="True" "RSTCOF 3" {
              frame False {
              }
              frame True {
                n2229 = property on="Electrical Contact Resistance ( % )" class="WFChart (strict)"("XScale.Minimum"=0.0 ("X Scale.Range:Minimum"), "XScale.Maximum"=600.0 ("X Scale.Range:Maximum"), "YScale.Minimum"=0.0 ("Y Scale.Range:Minimum"), "YScale.Maximum"=100.0 ("Y Scale.Range:Maximum")) -> ()  [unwired: 2 in, 2 out]
              }
            }
          }
        }
        n2230 = local read "RUN"() -> (w2887:bool)
        n2231 = case shown="False" w2887 {
          frame False {
          }
          frame True {
          }
        }
        n2232 = local read "RUN"() -> (w2891:bool)
        n2233 = case shown="False" w2891 {
          tunnel: [FALSE ("TEST RUNNING") TRUE ("TEST RUNNING")] -> w2890
          frame False {
            w2983 = 0.0 ("Flag")
            n2234 = local write "Elapsed time"(0.0 ("elapsedtime")) -> ()
            n2235 = local write "Time Remaining"(w2983) -> ()
            n2236 = local write "Flag"(w2983) -> ()
            n2237 = local write "Remaining Time"(w2983) -> ()
          }
          frame True {
            n2238 = local write "Flag"(10.0 ("Flag")) -> ()
          }
        }
        n2239 = local read "AIR TEMP"() -> (w2885:dbl)
        n2240 = Greater Or Equal?(x=w2885, y=15.0) -> (x >= y?=w2886:bool)
        "powstat" <- w2886
        n2241 = case shown="True" "Save & Continue" {
          frame False {
          }
          frame True {
            n2242 = local read "USER ID"() -> (w3291:string)
            n2243 = local read "FILE"() -> (w3299:string)
            n2244 = String Length(string=w3299) -> (length=w3297:i32)
            n2245 = String Length(string=w3291) -> (length=w3294:i32)
            n2246 = Greater?(x=w3297, y=0) -> (0:w3296:bool)
            n2247 = Greater?(x=w3294, y=0) -> (0:w3293:bool)
            n2248 = And(x=w3296, y=w3293) -> (x .and. y?=w3292:bool)
            n2249 = case shown="True" w3292 {
              frame False {
                n2250 = stacked-sequence {
                  frame #0 {
                    n2251 = One Button Dialog(message="Please Enter a File Name and Operator ID to save data !", button name ("OK")="Ok") -> ()  [unwired: 1 out]
                  }
                  frame #1 {
                    n2252 = local write "Save & Continue"(FALSE ("OK Button")) -> ()
                  }
                }
                n2253 = local write "Save & Continue"(FALSE ("OK Button")) -> ()
              }
              frame True {
                n2254 = stacked-sequence {
                  frame #0 {
                    n2255 = local read "FILE"() -> (w3305:string)
                    n2256 = call "file check.vi"("file name in"=w3305) -> ("file name out"=w3304:string)  [unwired: 9 in, 1 out]
                    n2257 = call <vilib>:"Application Directory.vi"() -> ("Application Directory"=w3315:path)
                    n2258 = Build Path(base path=w3315, name or relative path="data") -> (appended path=w3314:path)
                    n2259 = call <vilib>:"Trim Whitespace.vi"("string"=w3304) -> ("trimmed string"=w3312:string)  [unwired: 1 in]
                    n2260 = call <vilib>:"Trim Whitespace.vi"("string"=w3304) -> ("trimmed string"=w3313:string)  [unwired: 1 in]
                    n2261 = List Folder(path=w3314) -> (folder names=w3310:string[])  [unwired: 3 in, 3 out]
                    n2262 = Match Pattern(string=w3312, regular expression="_(") -> (before substring=w3309:string)  [unwired: 1 in, 3 out]
                    n2263 = for {
                      tunnel: w3310 -> [w3324] mode=indexing
                      tunnel: w3309 -> [w3322]
                      shift-right: [w3320] -> w3307
                      shift-left: bool[] [] -> [w3321]
                      n2264 = Match Pattern(string=w3324, regular expression="_(") -> (before substring=w3323:string)  [unwired: 1 in, 3 out]
                      n2265 = Equal?(x=w3323, y=w3322) -> (x = y?=w3319:bool)
                      n2266 = case shown="True" w3319 {
                        tunnel: w3319 -> [_ w3327]
                        tunnel: w3321 -> [w3326 w3329]
                        tunnel: [w3326 w3328] -> w3320
                        frame False {
                        }
                        frame True {
                          n2267 = Insert Into Array(array=w3329, new element=w3327) -> (w3328:bool[])  [unwired: 1 in]
                        }
                      }
                    }
                    n2268 = Equal?(x=w3310, y=w3309) -> (x = y?=w3318:bool[])
                    n2269 = Or Array Elements(Boolean array=w3318) -> (logical OR=w3317:bool)
                    n2270 = Array Size(array=w3307) -> (size(s)=w3306:i32)
                    n2271 = case shown="True" w3317 {
                      tunnel: w3313 -> [_ w3337]
                      tunnel: w3306 -> [_ w3330]
                      frame False {
                      }
                      frame True {
                        n2272 = Number To Decimal String(number=w3330) -> (decimal integer string=w3333:string)  [unwired: 1 in]
                        n2273 = Search/Split String(string=w3337, search string/char (-)="_(" ("regular expression")) -> (substring before match=w3335:string)  [unwired: 1 in, 2 out]
                        n2274 = Concatenate Strings(w3335, "_(" ("regular expression"), w3333, ")" ("regular expression")) -> (w3331:string)
                        n2275 = local write "FILE"(w3331) -> ()
                      }
                    }
                  }
                  frame #1 {
                    w3340 = 0.0
                    w3353 = cluster{"y":dbl, dbl, "y":dbl}[] [] ("History Data")
                    w3354 = FALSE ("Heater Button")
                    (unwired) ")!" ("string")
                    (unwired) ")" ("string")
                    w3352 = dbl[] [] ("History Data")
                    w3358 = "\r"
                    # "C:\\WinDucom\\Data\\"
                    # "C:\\LAB-IQ-NXT\\data"
                    n2276 = local write "Humidity ( %RH )"(w3340) -> ()
                    n2277 = local write "Frequency ( Hz )"(w3340) -> ()
                    n2278 = local write "Stroke 3"(w3340) -> ()
                    n2279 = local write "speedop"(0.0 ("PIDclk 2")) -> ()
                    n2280 = local write "Set Temp 2"(65.0 ("Set Temp 2")) -> ()
                    n2281 = local write "AIR TEMP"(w3340) -> ()
                    n2282 = local write "clk"(0.0 ("clk")) -> ()
                    n2283 = local write "Stroke 4"(w3340) -> ()
                    n2284 = local write "COF 2"(w3340) -> ()
                    n2285 = local write "TEMP"(w3340) -> ()
                    n2286 = local write "ecr 3"(w3340) -> ()
                    n2287 = local write "FF 3"(w3340) -> ()
                    n2288 = local write "FF 2"(w3340) -> ()
                    n2289 = property on="Humidity ( %RH ) 2" class="WFChart (strict)"("History Data"=w3352) -> ()  [unwired: 2 in, 2 out]
                    n2290 = property on="Coefficient of Friction" class="WFChart (strict)"("History Data"=w3352) -> ()  [unwired: 2 in, 2 out]
                    n2291 = property on="Coefficient of Friction" class="WFChart (strict)"("History Data"=w3352) -> ()  [unwired: 2 in, 2 out]
                    n2292 = property on="Frictional Force ( N )" class="WFChart (strict)"("History Data"=w3352) -> ()  [unwired: 2 in, 2 out]
                    n2293 = property on="Electrical Contact Resistance ( % )" class="WFChart (strict)"("History Data"=w3352) -> ()  [unwired: 2 in, 2 out]
                    n2294 = property on="Electrical Contact Resistance ( % )" class="WFChart (strict)"("History Data"=w3352) -> ()  [unwired: 2 in, 2 out]
                    n2295 = property on="Temperature ( Deg C )" class="WFChart (strict)"("History Data"=w3352) -> ()  [unwired: 2 in, 2 out]
                    n2296 = property on="Frictional Force ( N )" class="WFChart (strict)"("History Data"=w3352) -> ()  [unwired: 2 in, 2 out]
                    n2297 = property on="Coefficient of Friction" class="WFChart (strict)"("History Data"=w3352) -> ()  [unwired: 2 in, 2 out]
                    n2298 = property on="Frictional Force ( N )" class="WFChart (strict)"("History Data"=w3352) -> ()  [unwired: 2 in, 2 out]
                    n2299 = property on="Electrical Contact Resistance ( % )" class="WFChart (strict)"("History Data"=w3352) -> ()  [unwired: 2 in, 2 out]
                    n2300 = property on="Temperature ( Deg C )" class="WFChart (strict)"("History Data"=w3352) -> ()  [unwired: 2 in, 2 out]
                    n2301 = property on="Stroke ( mm )" class="WFChart (strict)"("History Data"=w3353) -> ()  [unwired: 2 in, 2 out]
                    n2302 = property on="Stroke ( mm )" class="WFChart (strict)"("History Data"=w3353) -> ()  [unwired: 2 in, 2 out]
                    n2303 = local write "Humidity"(w3354) -> ()
                    n2304 = local write "Heater Button"(w3354) -> ()
                    n2305 = local read "FILE"() -> (w3348:string)
                    n2306 = disable-structure shown="Enabled" {
                      disable-tunnel: [w3392 _] -> w3339
                      frame Enabled {
                        n2307 = local read "NORMAL LOAD"() -> (w3392:dbl)
                      }
                      frame Disabled {
                      }
                    }
                    n2308 = call "file check.vi"("file name in"=w3348) -> ("error out"=w3351:errorcluster, "file name out"=w3345:string)  [unwired: 9 in]
                    n2309 = call "FILE PATH CREATION.vi"("error in"=w3351, "FILE NAME :"=w3345) -> ("FILE OUT"=w3344:path)  [unwired: 8 in, 1 out]
                    n2310 = Concatenate Strings(w3345, ".dgf" ("Substring")) -> (w3350:string)
                    n2311 = Concatenate Strings(w3345, ".duf" ("Substring")) -> (w3346:string)
                    n2312 = Multiply(x=w3339, y=1.0) -> (x*y=w3371:dbl)
                    n2313 = Build Path(base path=w3344, name or relative path=w3350) -> (appended path=w3343:path)
                    n2314 = Build Path(base path=w3344, name or relative path=w3346) -> (appended path=w3342:path)
                    n2315 = Number To Fractional String(number=w3371, width (-)=i16 5, precision (6)=i16 2) -> (F-format string=w3379:string)  [unwired: 1 in]
                    n2316 = local read "tested by"() -> (w3338:string)
                    n2317 = local read "Fuel Discription :"() -> (w3367:string)
                    n2318 = local read "Batch Ref Num :"() -> (w3356:string)
                    n2319 = Get Date/Time String(date format (0)=enum16{"short", "long", "abbreviated"}."short") -> (date string=w3390:string, time string=w3387:string)  [unwired: 2 in]
                    n2320 = local read "Remarks :"() -> (w3366:string)
                    n2321 = Concatenate Strings("Load :- " ("Substring"), w3379, " grams ," ("Substring")) -> (w3378:string)
                    n2322 = local read "String 41"() -> (w3359:string)
                    n2323 = Concatenate Strings(w3367) -> (w3368:string)
                    n2324 = Concatenate Strings(w3356) -> (w3355:string)
                    n2325 = Concatenate Strings(w3338) -> (w3362:string)
                    n2326 = Concatenate Strings("(" ("Substring"), w3390, ")" ("Substring"), w3387) -> (w3361:string)
                    "concatenated string" <- w3361
                    n2327 = Concatenate Strings(w3366, "," ("string")) -> (w3365:string)
                    n2328 = Concatenate Strings("  TIME;      COF;       STROKE;     AIR TEMP;  TEMP;  HUMIDITY;  ECR; PID-OUT; FREQUENCY" ("Substring"), "\r") -> (w3374:string)
                    n2329 = Concatenate Strings(w3359, w3358, "Fuel Discription :-" ("Substring"), w3368, w3358, w3378, w3358, "Batch Ref Num :-" ("Substring"), w3355, w3358, " Remarks :- " ("Substring"), w3365, w3358, " Date :- " ("Substring"), w3361, w3358, "Tested By :-" ("Substring"), w3362) -> (w3372:string)
                    "REMARKS" <- w3372
                    n2330 = call <vilib>:"Write Characters To File.vi"("append to file? (new file:F)"=FALSE, "character string"=w3374, "file path (dialog if empty)"=w3343) -> ()  [unwired: 2 in, 1 out]
                    n2331 = call <vilib>:"Write Characters To File.vi"("append to file? (new file:F)"=FALSE, "character string"=w3372, "file path (dialog if empty)"=w3342) -> ()  [unwired: 2 in, 1 out]
                  }
                  frame #2 {
                    n2332 = local write "Cycles elapsed"(0 ("Cycles elapsed")) -> ()
                    n2333 = local write "cyclecount"(0 ("cyclecount")) -> ()
                    n2334 = local write "Save & Continue"(FALSE ("OK")) -> ()
                    n2335 = local write "autostrtflg"(TRUE ("autostrtflg")) -> ()
                    n2336 = local write "Save"(FALSE ("Save")) -> ()
                    n2337 = Get Date/Time In Seconds() -> (seconds since 1Jan1904=w3397:timestamp)
                    n2338 = To Double Precision Float(number=w3397) -> (double precision float=w3396:dbl)
                    n2339 = local write "acq timer"(w3396) -> ()
                    n2340 = One Button Dialog(message="Please ensure sample is mounted properly and machine is ready in all aspects for testing !", button name ("OK")="Ok") -> ()  [unwired: 1 out]
                  }
                  frame #3 {
                    n2341 = stacked-sequence {
                      frame #0 {
                        n2342 = local write "Main Dashboard Buttons"(T1."Dashboard" ("Main Dashboard Buttons")) -> ()
                        n2343 = local write "Main Tab"(T2."Acquire" ("Main Tab")) -> ()
                      }
                      frame #1 {
                        n2344 = local write "EVENT LOG"("" ("EVENT LOG")) -> ()
                      }
                      frame #2 {
                        n2345 = Wait (ms)(milliseconds to wait=u32 50) -> ()  [unwired: 1 out]
                      }
                      frame #3 {
                        n2346 = disable-structure shown="Disabled" {
                          frame Disabled {
                            n2347 = local read "EVENT LOG"() -> (w3409:string)
                            n2348 = call "Event Log.vi"("Content"="Test Details", "EVENT LOG"=w3409) -> ("EVENT LOG"=w3408:string)  [unwired: 8 in, 1 out]
                            n2349 = local write "EVENT LOG"(w3408) -> ()
                          }
                          frame Enabled {
                          }
                        }
                      }
                      frame #4 {
                        n2350 = Wait (ms)(milliseconds to wait=u32 50) -> ()  [unwired: 1 out]
                      }
                      frame #5 {
                        n2351 = local read "FILE"() -> (w3411:string)
                        n2352 = Concatenate Strings("File Name :" ("Content"), w3411) -> (w3412:string)
                        n2353 = local read "EVENT LOG"() -> (w3415:string)
                        n2354 = call "Event Log.vi"("Content"=w3412, "EVENT LOG"=w3415) -> ("EVENT LOG"=w3414:string)  [unwired: 8 in, 1 out]
                        n2355 = local write "EVENT LOG"(w3414) -> ()
                      }
                      frame #6 {
                        n2356 = Wait (ms)(milliseconds to wait=u32 50) -> ()  [unwired: 1 out]
                      }
                      frame #7 {
                        n2357 = local read "Batch Ref Num :"() -> (w3417:string)
                        n2358 = Concatenate Strings("Batch Ref No :" ("Content"), w3417) -> (w3418:string)
                        n2359 = local read "EVENT LOG"() -> (w3421:string)
                        n2360 = call "Event Log.vi"("Content"=w3418, "EVENT LOG"=w3421) -> ("EVENT LOG"=w3420:string)  [unwired: 8 in, 1 out]
                        n2361 = local write "EVENT LOG"(w3420) -> ()
                      }
                      frame #8 {
                        n2362 = Wait (ms)(milliseconds to wait=u32 50) -> ()  [unwired: 1 out]
                      }
                      frame #9 {
                        n2363 = local read "tested by"() -> (w3423:string)
                        n2364 = Concatenate Strings("Tested By :" ("Content"), w3423) -> (w3424:string)
                        n2365 = local read "EVENT LOG"() -> (w3427:string)
                        n2366 = call "Event Log.vi"("Content"=w3424, "EVENT LOG"=w3427) -> ("EVENT LOG"=w3426:string)  [unwired: 8 in, 1 out]
                        n2367 = local write "EVENT LOG"(w3426) -> ()
                      }
                      frame #10 {
                        n2368 = Wait (ms)(milliseconds to wait=u32 50) -> ()  [unwired: 1 out]
                      }
                      frame #11 {
                        n2369 = local read "TEST STANDARD"() -> (w3430:T3)
                        n2370 = case shown="\"ASTM D6079\", Default" w3430 {
                          tunnel: ["ASTM D6079" "ISO 12156" "CEC F-096-A-06" "Custom"] -> w3429
                          frame "ASTM D6079", Default {
                          }
                          frame "ISO 12156" {
                          }
                          frame "CEC F-096-A-06" {
                          }
                          frame "Custom" {
                          }
                        }
                        n2371 = Concatenate Strings("Test Standard :" ("Content"), w3429) -> (w3431:string)
                        n2372 = local read "EVENT LOG"() -> (w3434:string)
                        n2373 = call "Event Log.vi"("Content"=w3431, "EVENT LOG"=w3434) -> ("EVENT LOG"=w3433:string)  [unwired: 8 in, 1 out]
                        n2374 = local write "EVENT LOG"(w3433) -> ()
                      }
                      frame #12 {
                        n2375 = Wait (ms)(milliseconds to wait=u32 50) -> ()  [unwired: 1 out]
                      }
                      frame #13 {
                        n2376 = local read "Fuel Discription :"() -> (w3440:string)
                        n2377 = Concatenate Strings("Fuel Description :" ("Content"), w3440) -> (w3441:string)
                        n2378 = local read "EVENT LOG"() -> (w3444:string)
                        n2379 = call "Event Log.vi"("Content"=w3441, "EVENT LOG"=w3444) -> ("EVENT LOG"=w3443:string)  [unwired: 8 in, 1 out]
                        n2380 = local write "EVENT LOG"(w3443) -> ()
                      }
                      frame #14 {
                        n2381 = Wait (ms)(milliseconds to wait=u32 50) -> ()  [unwired: 1 out]
                      }
                      frame #15 {
                        n2382 = local read "Remarks :"() -> (w3446:string)
                        n2383 = Concatenate Strings("Remarks :" ("Content"), w3446) -> (w3447:string)
                        n2384 = local read "EVENT LOG"() -> (w3450:string)
                        n2385 = call "Event Log.vi"("Content"=w3447, "EVENT LOG"=w3450) -> ("EVENT LOG"=w3449:string)  [unwired: 8 in, 1 out]
                        n2386 = local write "EVENT LOG"(w3449) -> ()
                      }
                      frame #16 {
                        n2387 = Wait (ms)(milliseconds to wait=u32 50) -> ()  [unwired: 1 out]
                      }
                      frame #17 {
                        n2388 = local read "USER ID"() -> (w3452:string)
                        n2389 = Concatenate Strings("Operator ID :" ("Content"), w3452) -> (w3454:string)
                        n2390 = local read "EVENT LOG"() -> (w3456:string)
                        n2391 = call "Event Log.vi"("Content"=w3454, "EVENT LOG"=w3456) -> ("EVENT LOG"=w3455:string)  [unwired: 8 in, 1 out]
                        n2392 = local write "EVENT LOG"(w3455) -> ()
                      }
                      frame #18 {
                        n2393 = Wait (ms)(milliseconds to wait=u32 50) -> ()  [unwired: 1 out]
                      }
                      frame #19 {
                        n2394 = disable-structure shown="Disabled" {
                          frame Disabled {
                            n2395 = local read "EVENT LOG"() -> (w3460:string)
                            n2396 = call "Event Log.vi"("Content"="Test Parameter", "EVENT LOG"=w3460) -> ("EVENT LOG"=w3459:string)  [unwired: 8 in, 1 out]
                            n2397 = local write "EVENT LOG"(w3459) -> ()
                          }
                          frame Enabled {
                          }
                        }
                      }
                      frame #20 {
                        n2398 = Wait (ms)(milliseconds to wait=u32 50) -> ()  [unwired: 1 out]
                      }
                      frame #21 {
                        n2399 = local read "Set Hz"() -> (w3464:dbl)
                        n2400 = Number To Fractional String(number=w3464, precision (6)=i16 2) -> (F-format string=w3463:string)  [unwired: 2 in]
                        n2401 = Concatenate Strings("Set Frequency [Hz] :" ("Content"), w3463) -> (w3466:string)
                        n2402 = local read "EVENT LOG"() -> (w3468:string)
                        n2403 = call "Event Log.vi"("Content"=w3466, "EVENT LOG"=w3468) -> ("EVENT LOG"=w3467:string)  [unwired: 8 in, 1 out]
